vi "Butterfly XY Graph.vi"() -> ()   [LabVIEW 2012]
uses:
  <vilib>/gmath/NI_Gmath.lvlib
panel:
  in  "radius as function of angle":string="exp(cos(t))-2*cos(4*t)+sin(t/12)^5" caption="极径（极角的函数）"
  in  "number of points":u32=2000 caption="点数"
  in  "end":dbl=45.0 caption="结束" format="%.2f"
  in  "start":dbl caption="开始" format="%.2f"
  out "Butterfly  Graph":T1(graph)
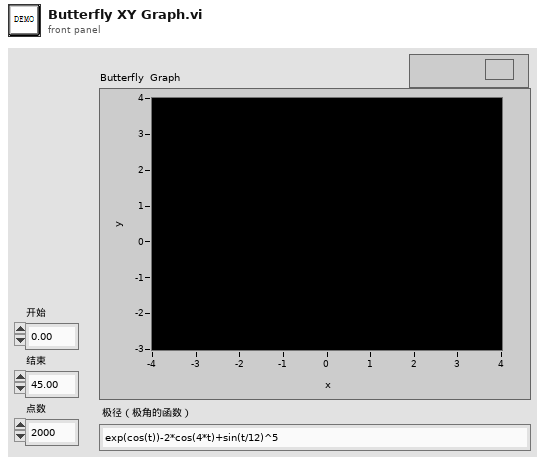
[diagram p1: front panel]
types:
  T1 = cluster{"Sinusoidal Pattern":dbl[], "Sinusoidal Pattern":dbl[]}
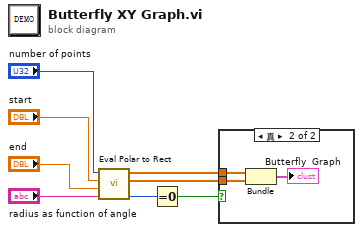
[diagram p0: block diagram]
diagram:
  n1 = call <vilib>:"Eval Polar to Rect.vi"("radius as function of angle"="radius as function of angle", "end"="end", "start"="start", "number of points"="number of points") -> ("error"=w2:i32, "Y"=w4:dbl[], "X"=w6:dbl[])  [unwired: 1 out]
  n2 = Equal To 0?(x=w2) -> (x = 0?=w1:bool)
  n3 = case shown="真" w1 {
    tunnel: w6 -> [_ w11]
    tunnel: w4 -> [_ w9]
    frame False {
    }
    frame True {
      n4 = Bundle("X"=w11, "Y"=w9) -> (→"Butterfly  Graph":cluster{"X":dbl[], "Y":dbl[]})  [unwired: 1 in]
    }
  }
